vi "PrintDisplay.vi"(8 "error in (no error)":errorcluster, 10 "InputStream":string, 11 "UserData":variant) -> (0 "error out":errorcluster)   [LabVIEW 2014]
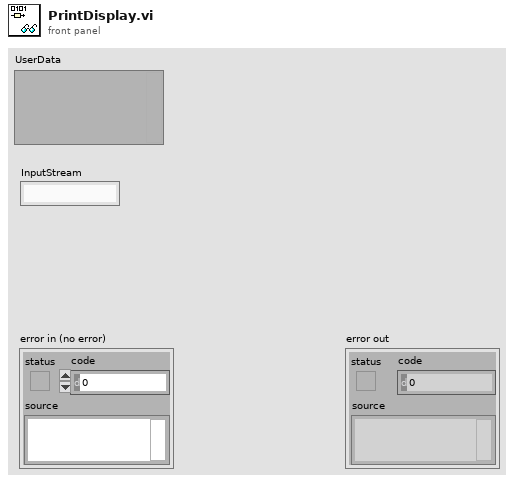
[diagram p1: front panel]
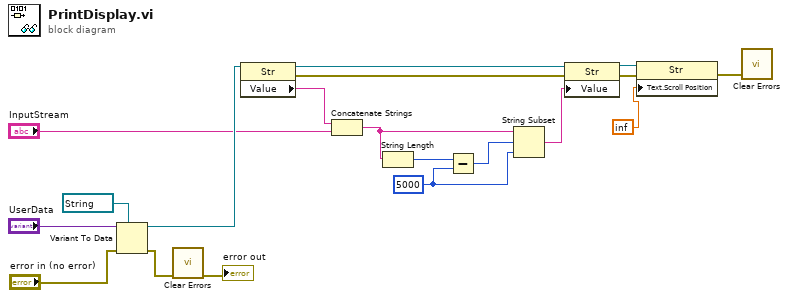
[diagram p0: block diagram]
diagram:
  w16 = 5000 ("y")
  n1 = Variant To Data(error in="error in (no error)", type=refnum<vi> refnum ("Output"), Variant="UserData") -> (data=w5:refnum<vi>, error out=w2:errorcluster)
  n2 = call <vilib>:"Clear Errors.vi"("error in (no error)"=w2) -> ("error out"=→"error out":errorcluster)  [unwired: 5 in, 1 out]
  n3 = property class="Str"(reference=w5) -> (reference out=w7:refnum<vi>, error out=w8:errorcluster, "Value"=w6:string)  [unwired: 1 in]
  n4 = Concatenate Strings(w6, "InputStream") -> (w13:string)
  n5 = String Length(string=w13) -> (length=w14:i32)
  n6 = Subtract(x=w14, y=w16) -> (x-y=w15:i32)
  n7 = String Subset(string=w13, offset (0)=w15, length (rest)=w16) -> (substring=w12:string)
  n8 = property class="Str"(reference=w7, error in=w8, "Value"=w12) -> (reference out=w10:refnum<vi>, error out=w9:errorcluster)
  n9 = property class="Str"(reference=w10, error in=w9, "Text.Scroll Position"=inf) -> (error out=w3:errorcluster)  [unwired: 1 out]
  n10 = call <vilib>:"Clear Errors.vi"("error in (no error)"=w3) -> ()  [unwired: 5 in, 2 out]
